vi "Calculate Rates.vi"(10 "Duration (s)":dbl, 11 "Event Counts":T1) -> (3 "Event Counts with Rate":T1)   [LabVIEW 2019, in "Muon Data Post-Processing.lvlib"]
uses:
  Post-Processing/Muon Data Post-Processing.lvlib
  Counts.ctl
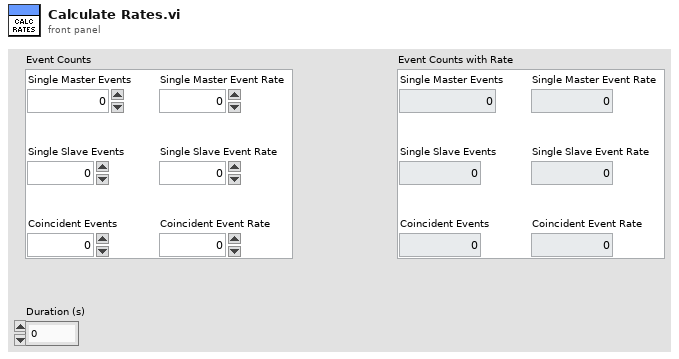
[diagram p1: front panel]
types:
  T1 = typedef "Counts.ctl" = cluster{"Single Master Events":i32, "Single Slave Events":i32, "Coincident Events":i32, "Single Master Event Rate":dbl, "Single Slave Event Rate":dbl, "Coincident Event Rate":dbl}
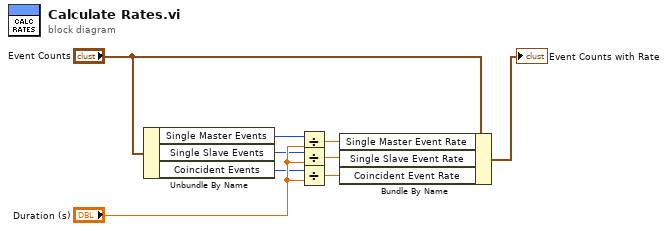
[diagram p0: block diagram]
diagram:
  n1 = Unbundle By Name("Event Counts") -> ("Single Master Events"=w6:i32, "Single Slave Events"=w5:i32, "Coincident Events"=w4:i32)
  n2 = Divide(x=w6, y="Duration (s)") -> (x/y=w3:dbl)
  n3 = Divide(x=w5, y="Duration (s)") -> (x/y=w2:dbl)
  n4 = Divide(x=w4, y="Duration (s)") -> (x/y=w1:dbl)
  n5 = Bundle By Name(cluster="Event Counts", "Single Master Event Rate"=w3, "Single Slave Event Rate"=w2, "Coincident Event Rate"=w1) -> (→"Event Counts with Rate":T1)
